vi "Handle UI events.vi"(8 "error in (no error)":errorcluster, 10 "Control in":refnum<vi>, 11 "String dropdown D Element in":refnum<class "String dropdown D Element.lvclass">) -> (0 "error out":errorcluster, 2 "Tabbed out?":bool, 3 "String dropdown D Element out":refnum<class "String dropdown D Element.lvclass">)   [LabVIEW 2018, in "D Datagrid Library.lvlib" / "String dropdown D Element.lvclass"]
doc: "Handles mousedown, keyboard, and other events. Override this VI if you want additional functionality for a specific element type."
uses:
  String dropdown D Element.lvclass
  <vilib>/event_ctls.llb/eventvkey.ctl
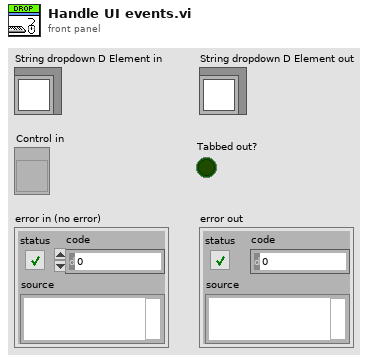
[diagram p1: front panel]
types:
  T1 = typedef "eventvkey.ctl" = enum16{"ASCII", "Enter", "Return", "Shift", "Ctrl", "Alt", "Cmd", "Opt", "Caps", "NumLock", "Clear", "Break", "Up", "Down", "Left", "Right", "Insert", "Delete", "Home", "End", "PageUp", "PageDown", "Escape", "Help", "Pause", "ScrollLock", "F1", "F2", "F3", "F4", "F5", "F6", "F7", "F8", "F9", "F10", "F11", "F12", "F13", "F14", "F15", "F16", "F17", "F18", "F19", "F20", "F21", "F22", "F23", "F24", "Play", "VolumeUp", "VolumeDown", "Mute", "Two Byte Char"}
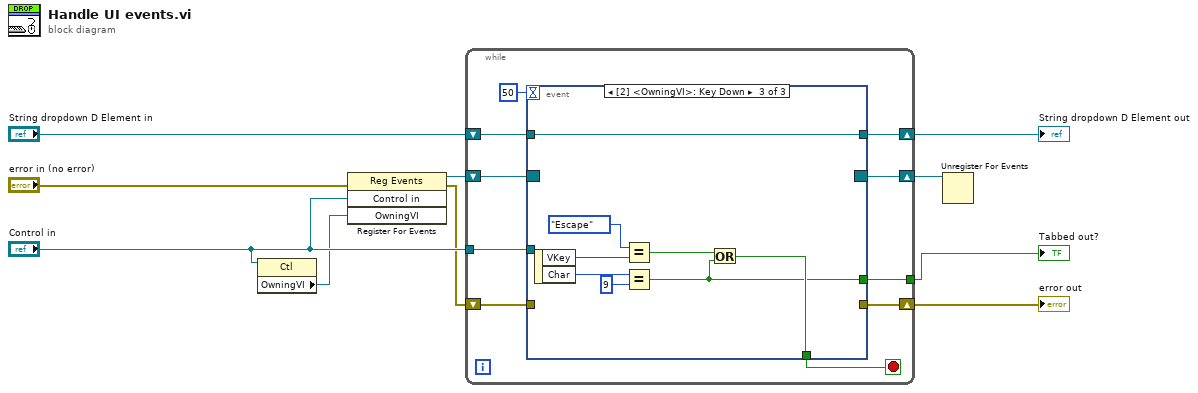
[diagram p0: block diagram]
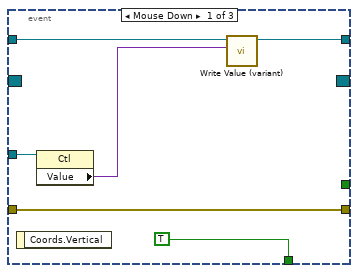
[diagram p2: hidden frame]
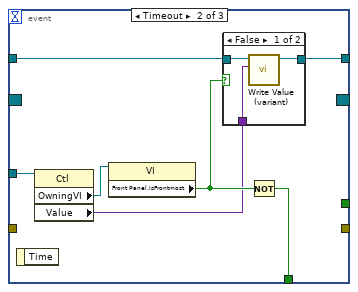
[diagram p3: hidden frame]
diagram:
  n1 = property class="Ctl"(reference="Control in") -> ("OwningVI"=w4:refnum<vi>)  [unwired: 1 in, 2 out]
  n2 = register-events(error in="error in (no error)", "Control in", w4) -> (reference out=w2:refnum<event-registration>, error out=w1:errorcluster)  [unwired: 1 in]
  n3 = while {
    shift-right: [w20] -> w9
    shift-left: "String dropdown D Element in" -> [w13]
    shift-right: [w18] -> w3
    shift-left: w2 -> [w19]
    shift-right: [w17] -> w8
    shift-left: w1 -> [w16]
    tunnel: "Control in" -> [w12]
    tunnel: [w11] -> w5
    stop <- w15 stop-if-true
    n4 = event shown="[2] <OwningVI>: Key Down" {
      selector: w19 -> [_ _ _]
      dyn-events: [_ _ _] -> w18
      timeout: 50 -> [_ _ _]
      tunnel: w13 -> [w24 w32 w42]
      tunnel: [w23 w31 w42] -> w20
      tunnel: [w26 _ _] -> w17
      tunnel: w16 -> [w26 _ _]
      tunnel: [TRUE w33 w39] -> w15
      tunnel: w12 -> [w22 w30 _]
      tunnel: [_ _ w38] -> w11
      event Mouse Down {
        n5 = event-data() -> ()  [unwired: 1 in, 1 out]
        n6 = property class="Ctl"(reference=w22) -> ("Value"=w21:variant)  [unwired: 1 in, 2 out]
        n7 = call-dynamic "Write Value (variant).vi"("Variant"=w21, "Ring D Element in"=w24) -> ("Ring D Element out"=w23:refnum<class "String dropdown D Element.lvclass">)  [unwired: 8 in, 1 out]
      }
      event Timeout {
        n8 = event-data() -> ()  [unwired: 1 in, 1 out]
        n9 = property class="Ctl"(reference=w30) -> ("OwningVI"=w29:refnum<vi>, "Value"=w27:variant)  [unwired: 1 in, 2 out]
        n10 = property class="VI"(reference=w29) -> ("Front Panel.IsFrontmost"=w28:bool)  [unwired: 1 in, 2 out]
        n11 = case shown="False" w28 {
          tunnel: w32 -> [w36 w37]
          tunnel: [w35 w37] -> w31
          tunnel: w27 -> [w34 _]
          frame False {
            n12 = call-dynamic "Write Value (variant).vi"("Variant"=w34, "Ring D Element in"=w36) -> ("Ring D Element out"=w35:refnum<class "String dropdown D Element.lvclass">)  [unwired: 8 in, 1 out]
          }
          frame True {
          }
        }
        n13 = Not(x=w28) -> (.not. x?=w33:bool)
      }
      event Key Down {
        n14 = event-data() -> ("VKey"=w45:T1, "Char"=w41:i16)  [unwired: 1 in]
        n15 = Equal?(x=eventvkey."Escape" ("VKey"), y=w45) -> (x = y?=w43:bool)
        n16 = Equal?(x=w41, y=i16 9) -> (x = y?=w38:bool)
        n17 = Or(x=w43, y=w38) -> (x .or. y?=w39:bool)
      }
    }
  }
  "String dropdown D Element out" <- w9
  "error out" <- w8
  "Tabbed out?" <- w5
  n18 = Unregister For Events(event registration refnum=w3) -> ()  [unwired: 1 in, 1 out]
